vi "read line log.vi"(2 "Line":i32=15, 3 "All Info":T1(array[cluster])=[[{"Port"=0, "Line"=0, "Description"="Move cart; TTL high = sci. cell (low = coll. cell)", "Default"=FALSE}, {"Port"=0, "Line"=1, "Description"="Rb on-resonant ODT light AOM; TTL high = on", "Default"=FALSE}, {"Port"=0, "Line"=2, "Description"="< line unused >", "Default"=FALSE}, {"Port"=0, "Line"=3, "Description"="Shutter for pump, repump beams; TTL high = open", "Default"=FALSE}, {"Port"=0, "Line"=4, "Description"="K 260 MHz AOM;  TTL low=off", "Default"=FALSE}, {"Port"=0, "Line"=5, "Description"="K OP/probe switch;  TTL low = OP", "Default"=TRUE}, {"Port"=0, "Line"=6, "Description"="CCD camera external sync; TTL low = take a picture", "Default"=TRUE}, {"Port"=0, "Line"=7, "Description"="Rb probe AOM switch; TTL high = off", "Default"=TRUE}, {"Port"=0, "Line"=8, "Description"="Rb probe shutter; TTL high = open", "Default"=FALSE}, {"Port"=0, "Line"=9, "Description"="MOT light shutter;  TTL high = open", "Default"=TRUE}, {"Port"=0, "Line"=10, "Description"="CCD camera shutter; TTL high = open", "Default"=FALSE}, {"Port"=0, "Line"=11, "Description"="YIG MUX; high=CMOT, low=MOT", "Default"=FALSE}, {"Port"=0, "Line"=12, "Description"="(unused, was K trap freq. switch)", "Default"=FALSE}, {"Port"=0, "Line"=13, "Description"="K probe shutter; TTL high=open", "Default"=FALSE}, {"Port"=0, "Line"=14, "Description"="Rb ZP AOM; TTL high = off", "Default"=TRUE}, {"Port"=0, "Line"=15, "Description"="Second MOT shutter;  TTL high=open", "Default"=TRUE}], [{"Port"=1, "Line"=0, "Description"="Rb shutter (before TA); TTL high = open", "Default"=TRUE}, {"Port"=1, "Line"=1, "Description"="Master Switch for Coils; 1 on, 0 off", "Default"=TRUE}, {"Port"=1, "Line"=2, "Description"="IP bleed servo TTL", "Default"=FALSE}, {"Port"=1, "Line"=3, "Description"="IP bleed master switch TTL", "Default"=FALSE}, {"Port"=1, "Line"=4, "Description"="A1 for Control Voltage (A1low, A0high -> MOT; high,low -> Q; high,high -> var. input BNC; low, low ->  \"?\" pot)", "Default"=FALSE}, {"Port"=1, "Line"=5, "Description"="A0 for Control Voltage", "Default"=TRUE}, {"Port"=1, "Line"=6, "Description"="Master Switch to IP trap;  TTL high=on", "Default"=FALSE}, {"Port"=1, "Line"=7, "Description"="Switch for pump quantization; TTL high = pump", "Default"=FALSE}, {"Port"=1, "Line"=8, "Description"="SRS burst trigger", "Default"=FALSE}, {"Port"=1, "Line"=9, "Description"="switches collection cell quantization (high = on)", "Default"=FALSE}, {"Port"=1, "Line"=10, "Description"="< line unused >", "Default"=FALSE}, {"Port"=1, "Line"=11, "Description"="Sci Cell Probe Quantization; TTL high = on", "Default"=FALSE}, {"Port"=1, "Line"=12, "Description"="U/D shim on the cart (TTL high=on)", "Default"=TRUE}, {"Port"=1, "Line"=13, "Description"="YIG control; TTL low=MOT/CMOT, high=maximum (for OP)", "Default"=FALSE}, {"Port"=1, "Line"=14, "Description"="IP bleed multiplex bit 1", "Default"=FALSE}, {"Port"=1, "Line"=15, "Description"="IP bleed multiplex bit 2", "Default"=FALSE}], [{"Port"=2, "Line"=0, "Description"="RF switch for K rf transfer", "Default"=FALSE}, {"Port"=2, "Line"=1, "Description"="flipper (high is z-axis probing)", "Default"=FALSE}, {"Port"=2, "Line"=2, "Description"="< line unused >", "Default"=FALSE}, {"Port"=2, "Line"=3, "Description"="Rb RP (vortex) AOM: TTL high = OP, low = CMOT", "Default"=TRUE}, {"Port"=2, "Line"=4, "Description"="Direction for cart coils; TTL high = anti-helmholtz, low = helmholtz", "Default"=TRUE}, {"Port"=2, "Line"=5, "Description"="< line unused >", "Default"=FALSE}, {"Port"=2, "Line"=6, "Description"="< line unused >", "Default"=FALSE}, {"Port"=2, "Line"=7, "Description"="< line unused >", "Default"=FALSE}, {"Port"=2, "Line"=8, "Description"="< line unused >", "Default"=FALSE}, {"Port"=2, "Line"=9, "Description"="< line unused >", "Default"=FALSE}, {"Port"=2, "Line"=10, "Description"="N/S shim cart (for bias field); TTL high = on", "Default"=FALSE}, {"Port"=2, "Line"=11, "Description"="< line unused >", "Default"=FALSE}, {"Port"=2, "Line"=12, "Description"="< line unused >", "Default"=FALSE}, {"Port"=2, "Line"=13, "Description"="< line unused >", "Default"=FALSE}, {"Port"=2, "Line"=14, "Description"="< line unused >", "Default"=FALSE}, {"Port"=2, "Line"=15, "Description"="< line unused >", "Default"=FALSE}], [{"Port"=3, "Line"=0, "Description"="N/S shim", "Default"=FALSE}, {"Port"=3, "Line"=1, "Description"="trigger for rf sweep (SRS GPIB address 13)", "Default"=FALSE}, {"Port"=3, "Line"=2, "Description"="< line unused >", "Default"=FALSE}, {"Port"=3, "Line"=3, "Description"="< line unused >", "Default"=FALSE}, {"Port"=3, "Line"=4, "Description"="YAG master control", "Default"=FALSE}, {"Port"=3, "Line"=5, "Description"="RF amp power", "Default"=TRUE}, {"Port"=3, "Line"=6, "Description"="< line unused >", "Default"=FALSE}, {"Port"=3, "Line"=7, "Description"="< line unused >", "Default"=FALSE}, {"Port"=3, "Line"=8, "Description"="rf switch for evaporation", "Default"=FALSE}, {"Port"=3, "Line"=9, "Description"="< line unused >", "Default"=FALSE}, {"Port"=3, "Line"=10, "Description"="< line unused >", "Default"=FALSE}, {"Port"=3, "Line"=11, "Description"="< line unused >", "Default"=FALSE}, {"Port"=3, "Line"=12, "Description"="< line unused >", "Default"=FALSE}, {"Port"=3, "Line"=13, "Description"="< line unused >", "Default"=FALSE}, {"Port"=3, "Line"=14, "Description"="< line unused >", "Default"=FALSE}, {"Port"=3, "Line"=15, "Description"="K trap frequency jump", "Default"=FALSE}]], 4 "Port":i32) -> (0 "Description":string="Second MOT shutter;  TTL high=open", 1 "Default  Value":bool=TRUE)   [LabVIEW 2017]
doc: "This subVI takes a TTL port (0-3) and line (0-15) and outputs a description and a default value for that TTL. This subVI need an input array that contains all the descriptions and default values. Get this array from \"line log (default values).vi\"."
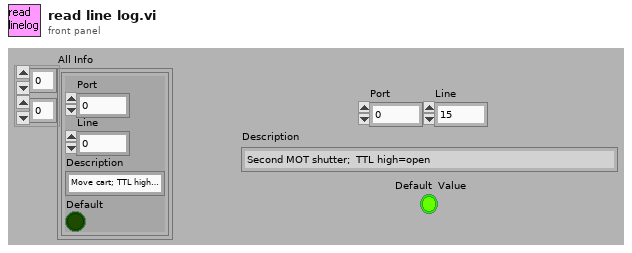
[diagram p1: front panel]
types:
  T1 = cluster{"Port":u32, "Line":u32, "Description":string, "Default":bool}[][]
  T2 = cluster{"Port":u32, "Line":u32, "Description":string, "Default":bool}
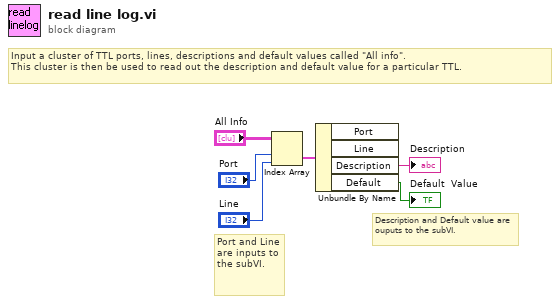
[diagram p0: block diagram]
diagram:
  # "Input a cluster of TTL ports, lines, descriptions and default values called \"All info\".\nThis cluster is then be used to read out the description and default value for a particular TTL."
  # "Description and Default value are ouputs to the subVI."
  # "Port and Line are inputs to the subVI."
  n1 = Index Array(array="All Info", index (row)="Port", index (col)="Line") -> (element=w3:T2)
  n2 = Unbundle By Name(w3) -> ("Description"=→"Description":string, "Default"=→"Default  Value":bool)  [unwired: 2 out]
